vi "Ramp SUBVI.vi"   [LabVIEW 2011]
types:
  T1 = cluster{"Driver Station Digital Input (1-8)[0]":bool, "Driver Station Digital Input (1-8)[1]":bool, "Driver Station Digital Input (1-8)[2]":bool, "Driver Station Digital Input (1-8)[3]":bool, "Driver Station Digital Input (1-8)[4]":bool, "Driver Station Digital Input (1-8)[5]":bool, "Driver Station Digital Input (1-8)[6]":bool, "Driver Station Digital Input (1-8)[7]":bool, "Driver Station Digital Input (1-8)[8]":bool}
  T2 = typedef "WPI_MotorControlDeviceRef.ctl" = cluster{"DeviceStatus":errorcluster, "Type":enum16{"PWM", "CAN"}, "PWM":cluster{"Digital Module":T3, "PWM Channel":T4, "DeadBand":T5}, "CAN":cluster{"Device Number":u8, "Control Mode":T6, "Semaphore":T7, "Max Vout":dbl}, "Invert":bool, "TransformRef":T8, "InvTransformRef":T8}
  T3 = typedef "FPGA_TypedefDigitalModule.ctl" = enum16{"Digital Module 1", "Digital Module 2"}
  T4 = typedef "FPGA_DIOPWMChannel.ctl" = enum8{"PWM 1", "PWM 2", "PWM 3", "PWM 4", "PWM 5", "PWM 6", "PWM 7", "PWM 8", "PWM 9", "PWM 10", "Invalid"}
  T5 = typedef "WPI_PWMDeadband.ctl" = cluster{"Name":string, "maxPositivePwm":i32, "minPositivePwm":i32, "centerPwm":i32, "maxNegativePwm":i32, "minNegativePwm":i32, "angularRange":u16}
  T6 = typedef "WPI_CANJaguar_ControlMode.ctl" = enum8{"Percent VBus", "Current", "Speed", "Position", "Voltage"}
  T7 = typedef "Semaphore RefNum" = refnum<k1>
  T8 = typedef "WPI_PWMTransform_ConPane.ctl" = refnum<vi>
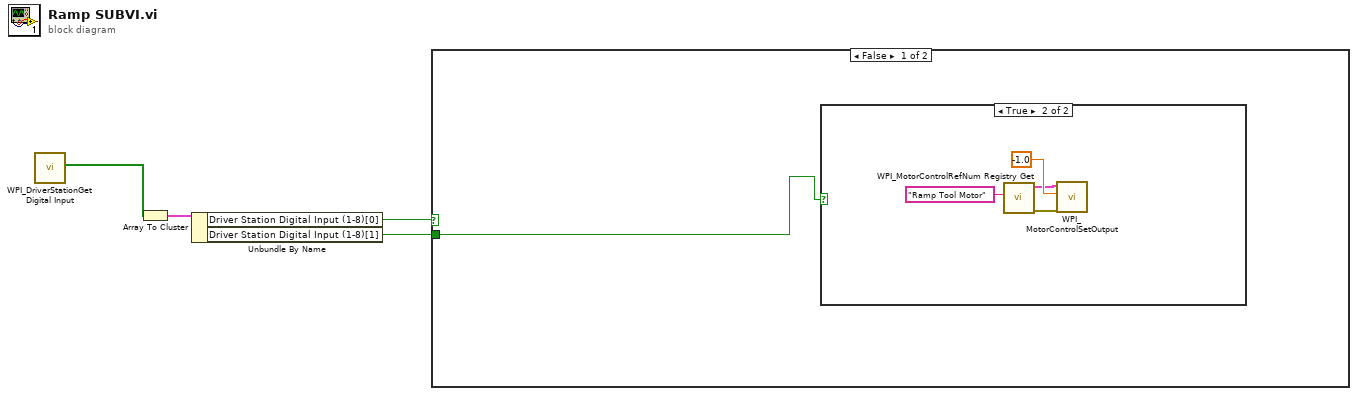
[diagram p0: block diagram]
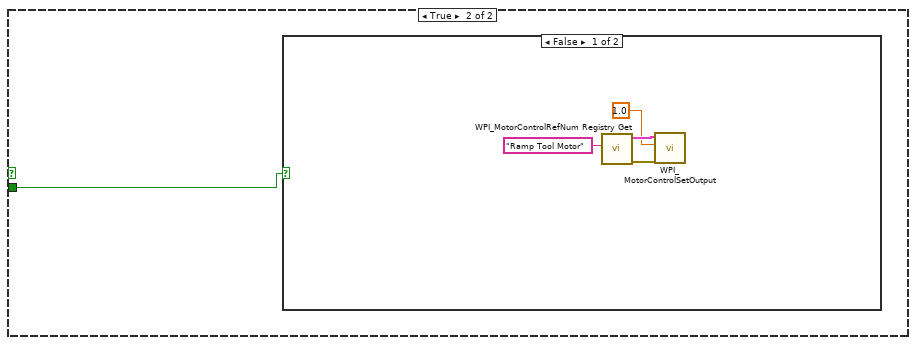
[diagram p3: hidden frame]
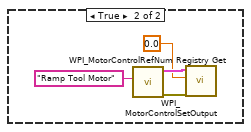
[diagram p4: hidden frame]
diagram:
  n1 = call <vilib>:"WPI_DriverStationGet Digital Input.vi"() -> ("Driver Station Digital Input (1-8)"=w2:bool[])  [unwired: 11 out]
  n2 = Array To Cluster(array=w2) -> (cluster=w4:T1)
  n3 = Unbundle By Name(w4) -> ("Driver Station Digital Input (1-8)[0]"=w3:bool, "Driver Station Digital Input (1-8)[1]"=w1:bool)
  n4 = case shown="False" w3 {
    tunnel: w1 -> [w5 w10]
    frame False {
      n5 = case shown="True" w5 {
        frame False {
        }
        frame True {
          n6 = call <vilib>:"WPI_MotorControlRefNum Registry Get.vi"("refnum name"="Ramp Tool Motor") -> ("error out"=w7:errorcluster, "MotorControlDevRef"=w6:T2)  [unwired: 9 in]
          n7 = call <vilib>:"WPI_MotorControlSetOutput.vi"("error in (no error)"=w7, "Output"=-1.0, "MotorControlDevRef"=w6) -> ()  [unwired: 7 in, 2 out]
        }
      }
    }
    frame True {
      n8 = case shown="False" w10 {
        frame False {
          n9 = call <vilib>:"WPI_MotorControlRefNum Registry Get.vi"("refnum name"="Ramp Tool Motor") -> ("error out"=w13:errorcluster, "MotorControlDevRef"=w14:T2)  [unwired: 9 in]
          n10 = call <vilib>:"WPI_MotorControlSetOutput.vi"("error in (no error)"=w13, "Output"=1.0, "MotorControlDevRef"=w14) -> ()  [unwired: 7 in, 2 out]
        }
        frame True {
          n11 = call <vilib>:"WPI_MotorControlRefNum Registry Get.vi"("refnum name"="Ramp Tool Motor") -> ("error out"=w17:errorcluster, "MotorControlDevRef"=w18:T2)  [unwired: 9 in]
          n12 = call <vilib>:"WPI_MotorControlSetOutput.vi"("error in (no error)"=w17, "Output"=0.0, "MotorControlDevRef"=w18) -> ()  [unwired: 7 in, 2 out]
        }
      }
    }
  }
